vi "吸光值读取.vi"(4 "error in (no error)":errorcluster caption="错误输入（无错误）", 6 "Container State":T3 caption="容器状态", 7 "Display State In":T2 caption="显示状态输入") -> (0 "error out":errorcluster caption="错误输出", 2 "Value":T1, 3 "Display State Out":T2 caption="显示状态输出")   [LabVIEW 2016, in "曲线模型.xctl"]
uses:
  <vilib>/_xctls/Container State.ctl
  <vilib>/_xctls/XControlSupport.lvlib
panel:
  # "将以下值显示控件替换为所需类型的显示控件。\n不要从连线板中删除该显示控件或其它显示控件。\n不要更改连线板模式。\n值显示控件应始终位于连线板输出端自顶部起第二个接线端。"
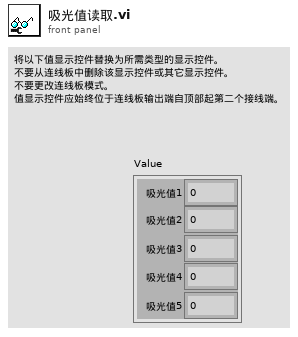
[diagram p1: front panel]
types:
  T1 = cluster{"Value":dbl, "Value 2":dbl, "Value 3":dbl, "Value 4":dbl, "Value 5":dbl}
  T2 = typedef "曲线模型.xctl/状态 1.ctl" = cluster{"模型选择":cluster{"参数":u8, "测量模式":u8, "量程":u8}, "吸光值":cluster{"Value":dbl, "Value 2":dbl, "Value 3":dbl, "Value 4":dbl, "Value 5":dbl}, "浓度":cluster{"标液浓度1":dbl, "标液浓度2":dbl, "标液浓度3":dbl, "标液浓度4":dbl, "标液浓度5":dbl}}
  T3 = typedef "XControlSupport.lvlib/Container State.ctl" = cluster{"Indicator?":bool, "Run Mode?":bool, " Refnum":refnum<vi>}
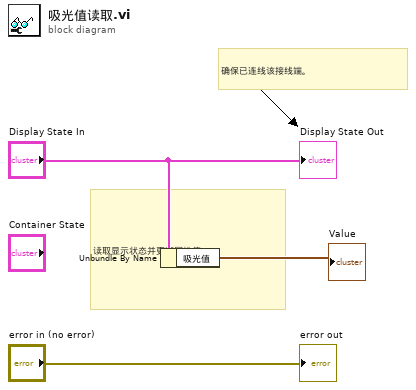
[diagram p0: block diagram]
diagram:
  # "确保已连线该接线端。"
  # "读取显示状态并更新属性值。"
  n1 = Unbundle By Name("Display State In") -> ("吸光值"=→"Value":T1)
  "error out" <- "error in (no error)"
  "Display State Out" <- "Display State In"
